vi "Day 2 - Cube Conundrum.vi"() -> ()   [LabVIEW 2020, in "AoC 2023.lvlib"]
uses:
  AoC 2023.lvlib
panel:
  out "Puzzle Part-2 Answer":string
  out "Puzzle Answer":string
  in  "Puzzle Input":string="Game 1: 3 blue, 4 red; 1 red, 2 green, 6 blue; 2 green\nGame 2: 1 blue, 2 green; 3 green, 4 blue, 1 red; 1 green, 1 blue\nGame 3: 8 green, 6 blue, 20 red; 5 blue, 4 red, 13 green; 5 green, 1 red\nGame 4: 1 green, 3 red, 6 blue; 3 green, 6 red; 3 green, 15 blue, 14 red\nGame 5: 6 red, 1 blue, 3 green; 2 blue, 1 red, 2 green"
  # "Enter the Puzzle Input and run the VI"
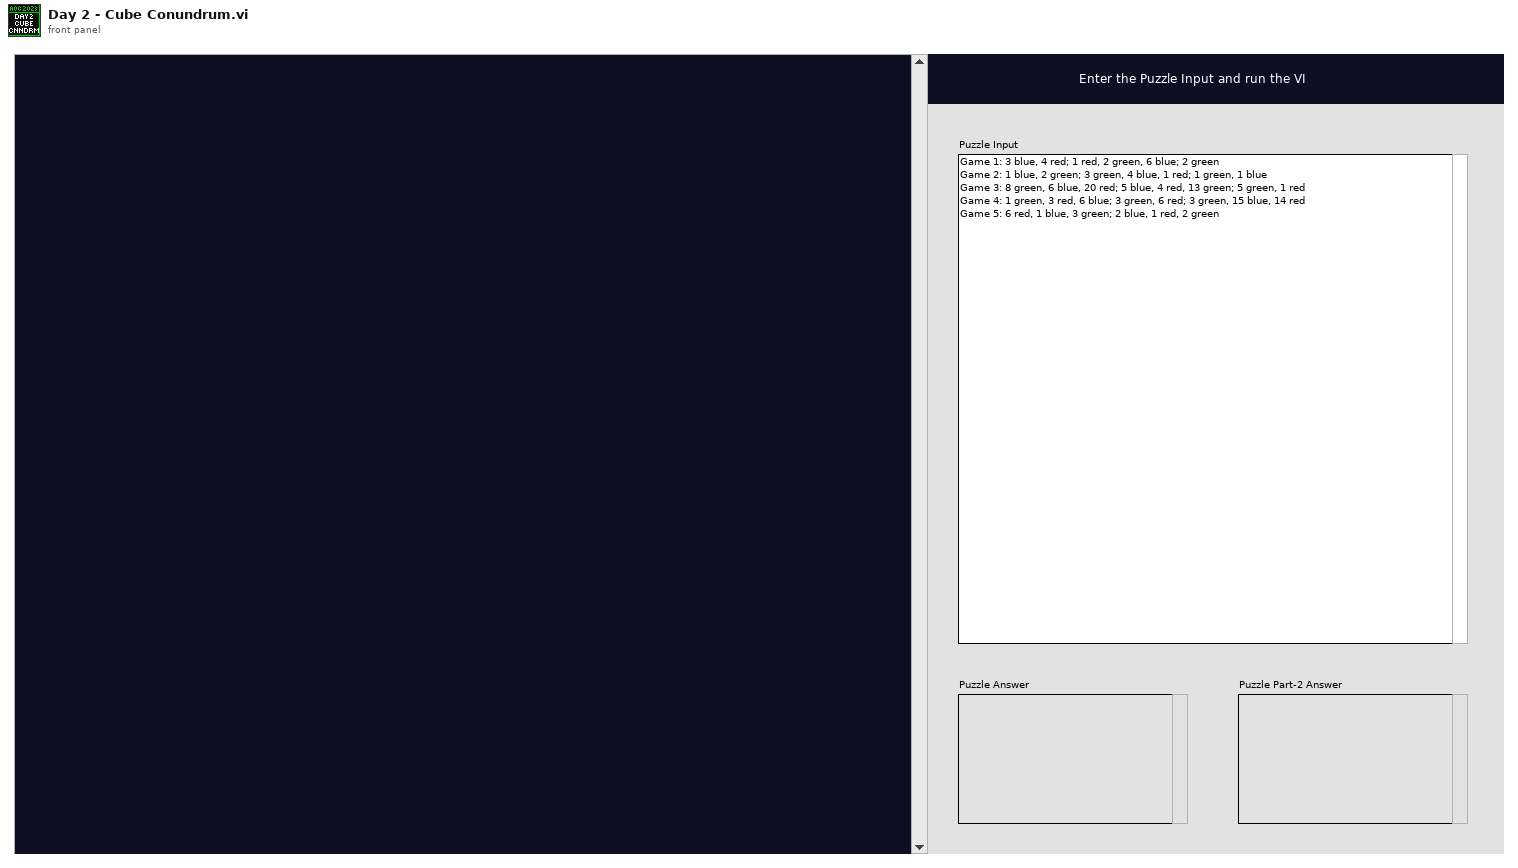
[diagram p1: front panel]
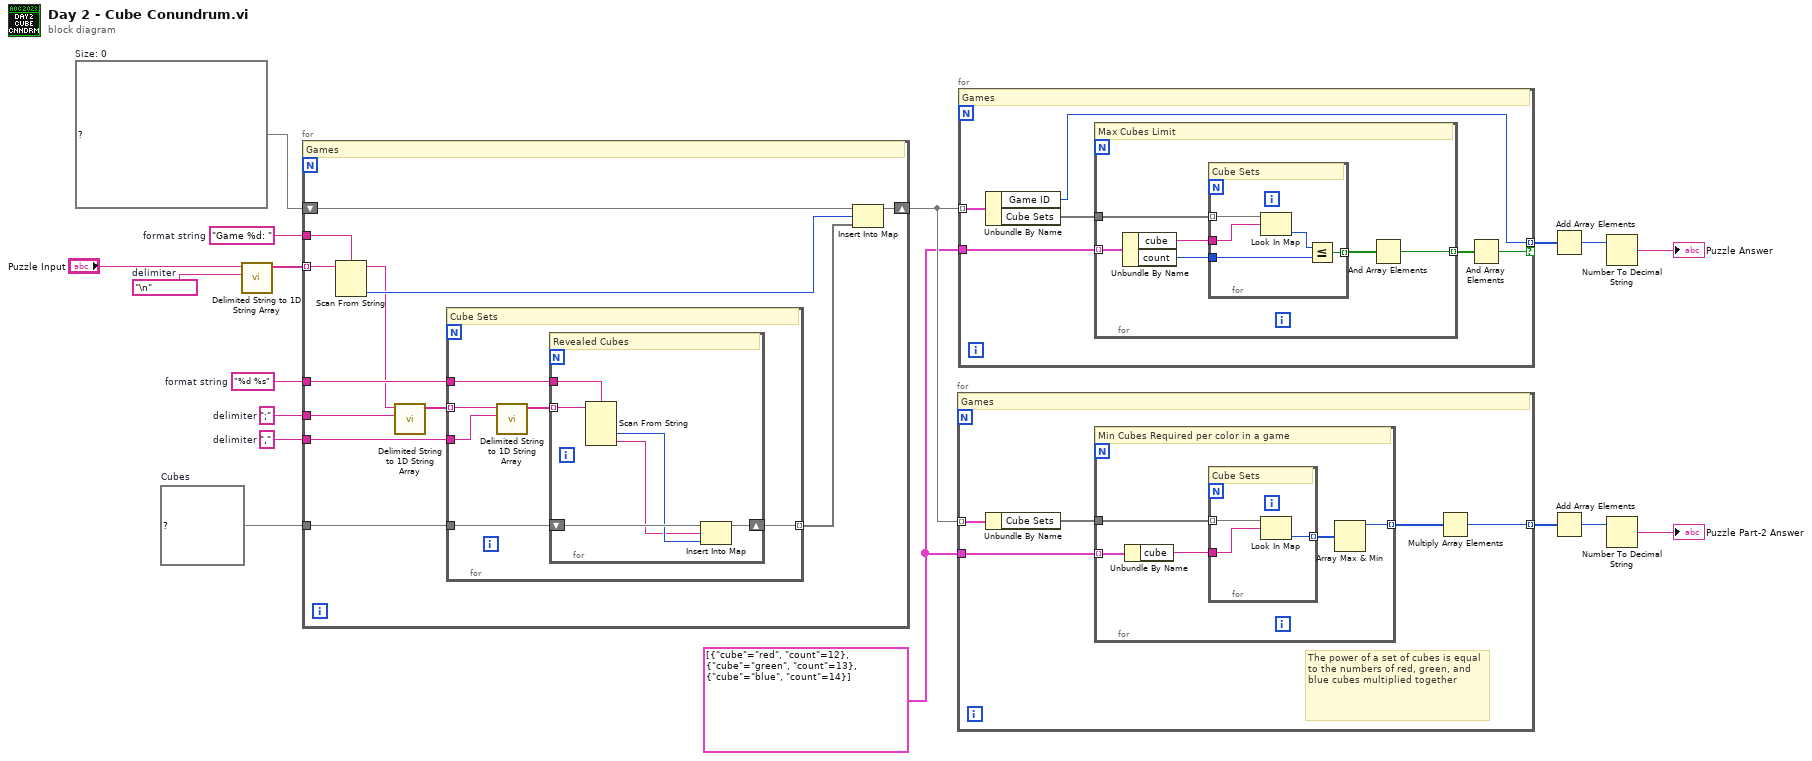
[diagram p0: block diagram]
diagram:
  w3 = cluster{"cube":string, "count":i32}[] [{"cube"="red", "count"=12}, {"cube"="green", "count"=13}, {"cube"="blue", "count"=14}]
  w7 = map{string, i32} {}  # Cubes
  w9 = ","  # delimiter
  w8 = ";"  # delimiter
  w10 = map{i32, map{string, i32}[]} {}  # Size: 0
  w14 = "%d %s"  # format string
  w15 = "Game %d: "  # format string
  w11 = "\n"  # delimiter
  n1 = call <vilib>:"Delimited String to 1D String Array.vi"("delimiter"=w11, "delimited string"="Puzzle Input") -> ("string array"=w12:string[])  [unwired: 9 in]
  n2 = for {
    tunnel: w12 -> [w29] mode=indexing
    tunnel: w15 -> [w28]
    shift-right: [w26] -> w4
    shift-left: w10 -> [w25]
    tunnel: w14 -> [w23]
    tunnel: w9 -> [w21]
    tunnel: w8 -> [w20]
    tunnel: w7 -> [w19]
    # "Games"
    n3 = Scan From String(format string=w28, input string=w29) -> (remaining string=w18:string, output 1=w27:i32)  [unwired: 3 in, 2 out]
    n4 = call <vilib>:"Delimited String to 1D String Array.vi"("delimiter"=w20, "delimited string"=w18) -> ("string array"=w24:string[])  [unwired: 9 in]
    n5 = for {
      tunnel: w24 -> [w35] mode=indexing
      tunnel: w23 -> [w33]
      tunnel: [w32] -> w22 mode=indexing
      tunnel: w21 -> [w31]
      tunnel: w19 -> [w30]
      # "Cube Sets"
      n6 = call <vilib>:"Delimited String to 1D String Array.vi"("delimiter"=w31, "delimited string"=w35) -> ("string array"=w34:string[])  [unwired: 9 in]
      n7 = for {
        tunnel: w34 -> [w41] mode=indexing
        tunnel: w33 -> [w40]
        shift-right: [w39] -> w32
        shift-left: w30 -> [w38]
        # "Revealed Cubes"
        n8 = Scan From String(format string=w40, input string=w41) -> (output 1=w37:i32, output 2=w36:string)  [unwired: 4 in, 3 out]
        n9 = Insert Into Map(map in=w38, key=w36, value=w37) -> (map out=w39:map{string, i32})  [unwired: 2 out]
      }
    }
    n10 = Insert Into Map(map in=w25, key=w27, value=w22) -> (map out=w26:map{i32, map{string, i32}[]})  [unwired: 2 out]
  }
  n11 = for {
    tunnel: w4 -> [w46] mode=indexing
    tunnel: w3 -> [w44]
    tunnel: [w42] -> w2 mode=indexing
    # "The power of a set of cubes is equal to the numbers of red, green, and blue cubes multiplied together"
    # "Games"
    n12 = Unbundle By Name(w46) -> ("Cube Sets"=w45:map{string, i32}[])
    n13 = for {
      tunnel: w45 -> [w51]
      tunnel: w44 -> [w50] mode=indexing
      tunnel: [w47] -> w43 mode=indexing
      # "Min Cubes Required per color in a game"
      n14 = Unbundle By Name(w50) -> ("cube"=w49:string)
      n15 = for {
        tunnel: w51 -> [w54] mode=indexing
        tunnel: w49 -> [w53]
        tunnel: [w52] -> w48 mode=indexing
        # "Cube Sets"
        n16 = Look In Map(map=w54, key=w53) -> (value=w52:i32)  [unwired: 1 in, 1 out]
      }
      n17 = Array Max & Min(array=w48) -> (max value=w47:i32)  [unwired: 3 out]
    }
    n18 = Multiply Array Elements(1:w43) -> (0:w42:i32)
  }
  n19 = for {
    tunnel: w4 -> [w60] mode=indexing
    tunnel: w3 -> [w58]
    tunnel: [w55] -> w6 mode=indexing if=w56
    # "Games"
    n20 = Unbundle By Name(w60) -> ("Game ID"=w55:i32, "Cube Sets"=w59:map{string, i32}[])
    n21 = for {
      tunnel: w59 -> [w66]
      tunnel: [w61] -> w57 mode=indexing
      tunnel: w58 -> [w65] mode=indexing
      # "Max Cubes Limit"
      n22 = Unbundle By Name(w65) -> ("cube"=w64:string, "count"=w63:i32)
      n23 = for {
        tunnel: w66 -> [w71] mode=indexing
        tunnel: w64 -> [w70]
        tunnel: w63 -> [w69]
        tunnel: [w67] -> w62 mode=indexing
        # "Cube Sets"
        n24 = Look In Map(map=w71, key=w70) -> (value=w68:i32)  [unwired: 1 in, 1 out]
        n25 = Less Or Equal?(x=w68, y=w69) -> (x <= y?=w67:bool)
      }
      n26 = And Array Elements(Boolean array=w62) -> (logical AND=w61:bool)
    }
    n27 = And Array Elements(Boolean array=w57) -> (logical AND=w56:bool)
  }
  n28 = Add Array Elements(numeric array=w6) -> (sum=w5:i32)
  n29 = Add Array Elements(numeric array=w2) -> (sum=w1:i32)
  n30 = Number To Decimal String(number=w5) -> (decimal integer string=→"Puzzle Answer":string)  [unwired: 1 in]
  n31 = Number To Decimal String(number=w1) -> (decimal integer string=→"Puzzle Part-2 Answer":string)  [unwired: 1 in]
